vi "Another VI week 2 Convert C to F.vi"() -> ()   [LabVIEW 2024]
panel:
  out "Deg F":dbl
  in  "Deg C":dbl
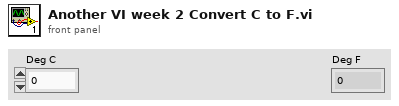
[diagram p1: front panel]
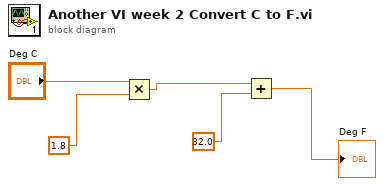
[diagram p0: block diagram]
diagram:
  n1 = Multiply(x="Deg C", y=1.8 ("x*y")) -> (x*y=w2:dbl)
  n2 = Add(x=w2, y=32.0) -> (x+y=→"Deg F":dbl)
